vi "Set Topic Actor.vi"(8 "error in (no error)":errorcluster, 10 "Topic Actor":refnum<class "Topic Actor.lvclass">, 11 "Message Broker in":refnum<class "Message Broker.lvclass">) -> (0 "error out":errorcluster, 3 "Message Broker out":refnum<class "Message Broker.lvclass">)   [LabVIEW 2016, in "Stream Mediator.lvlib" / "Message Broker.lvclass"]
doc: "--\nCopyright © 2017 Composed SystemsI All rights reserved.\n\nAuthor: Jon McBee <jon.mcbee@composed.io>\n\nThis library is provided \"AS IS\" ,WITHOUT WARRANTIES OR\nCONDITIONS OF ANY KIND, either express or implied.\n\nComposed Systems -- composed.io\n\nStream 0.0.1.1\nJon McBee - Composed Systems\nCopyright (c) 2017, Composed Systems"
uses:
  <userlib>/Composed Systems/Stream/Mediator/Classes/Message Broker/Message Broker.lvclass
  <userlib>/Composed Systems/Stream/Mediator/Classes/Topic Actor/Topic Actor.lvclass
  <userlib>/Composed Systems/Stream/Mediator/Classes/Message Broker/Message Broker.lvclass/Message Broker.ctl
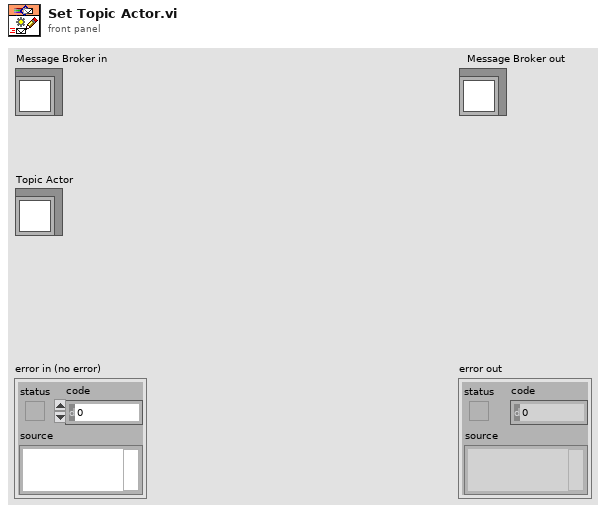
[diagram p1: front panel]
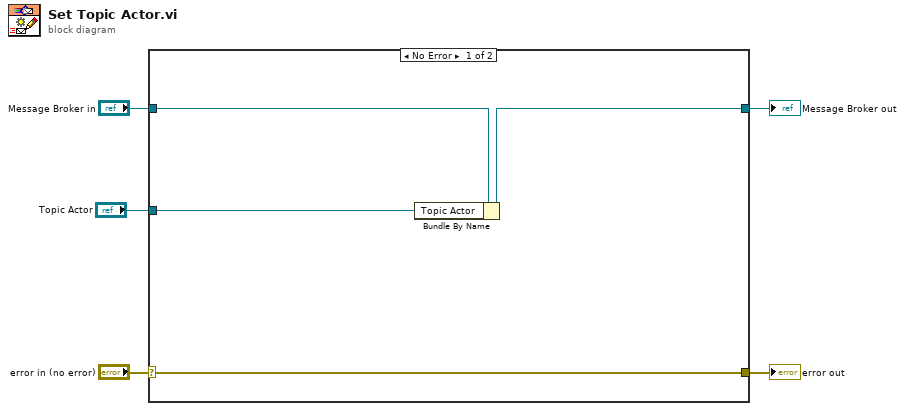
[diagram p0: block diagram]
diagram:
  n1 = case shown="No Error" "error in (no error)" {
    selector: "error in (no error)" -> [w9 w11]
    tunnel: [w9 w11] -> w4
    tunnel: [w7 w10] -> w2
    tunnel: "Message Broker in" -> [w8 w10]
    tunnel: "Topic Actor" -> [w6 _]
    frame No Error {
      n2 = Bundle By Name(cluster=w8, "Topic Actor"=w6) -> (w7:refnum<class "Message Broker.lvclass">)
    }
    frame Error {
    }
  }
  "error out" <- w4
  "Message Broker out" <- w2
